vi "DIO read.vi"(8 "error in (no error)":errorcluster, 11 "DIO in":refnum<class "DIO.lvclass">) -> (0 "error out":errorcluster, 2 "read":bool, 3 "DIO out":refnum<class "DIO.lvclass">)   [LabVIEW 2019, in "my FPGA lib.lvlib" / "DIO.lvclass"]
uses:
  DIO.lvclass
  DIO.lvclass/DIO.ctl
  <vilib>/Utility/error.llb/Error Cluster From Error Code.vi
  <vilib>/rvi/errors/niLvFpgaAdjustHostInterfaceError.vi
  <vilib>/rvi/interface/nirviReadWriteControl/nirviReadWriteControl.xnode
  NiFpgaLv.dll
  <vilib>/rvi/interface/Simulation/niFpgaSimulationCallBeginRW.vi
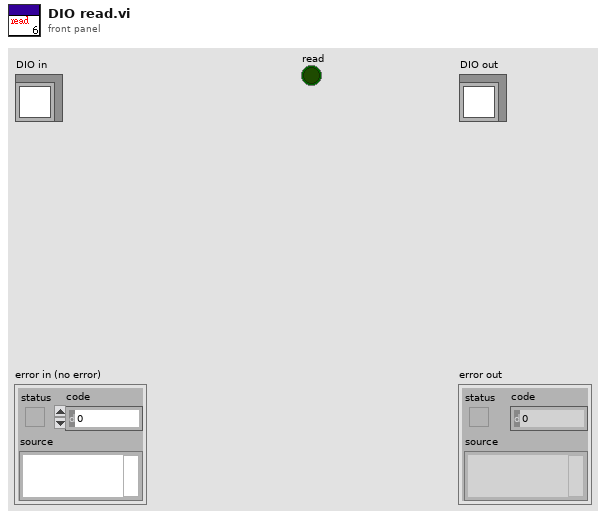
[diagram p1: front panel]
types:
  T1 = typedef "my FPGA lib.lvlib/DIO.lvclass/DIO enum.ctl" = enum16{"US.1", "US.2", "US.3", "US.4", "H.1", "H.2", "H.3", "H.4", "H.5"}
  T2 = typedef "my FPGA lib.lvlib/DIO.lvclass/port.ctl" = enum16{"US", "H."}
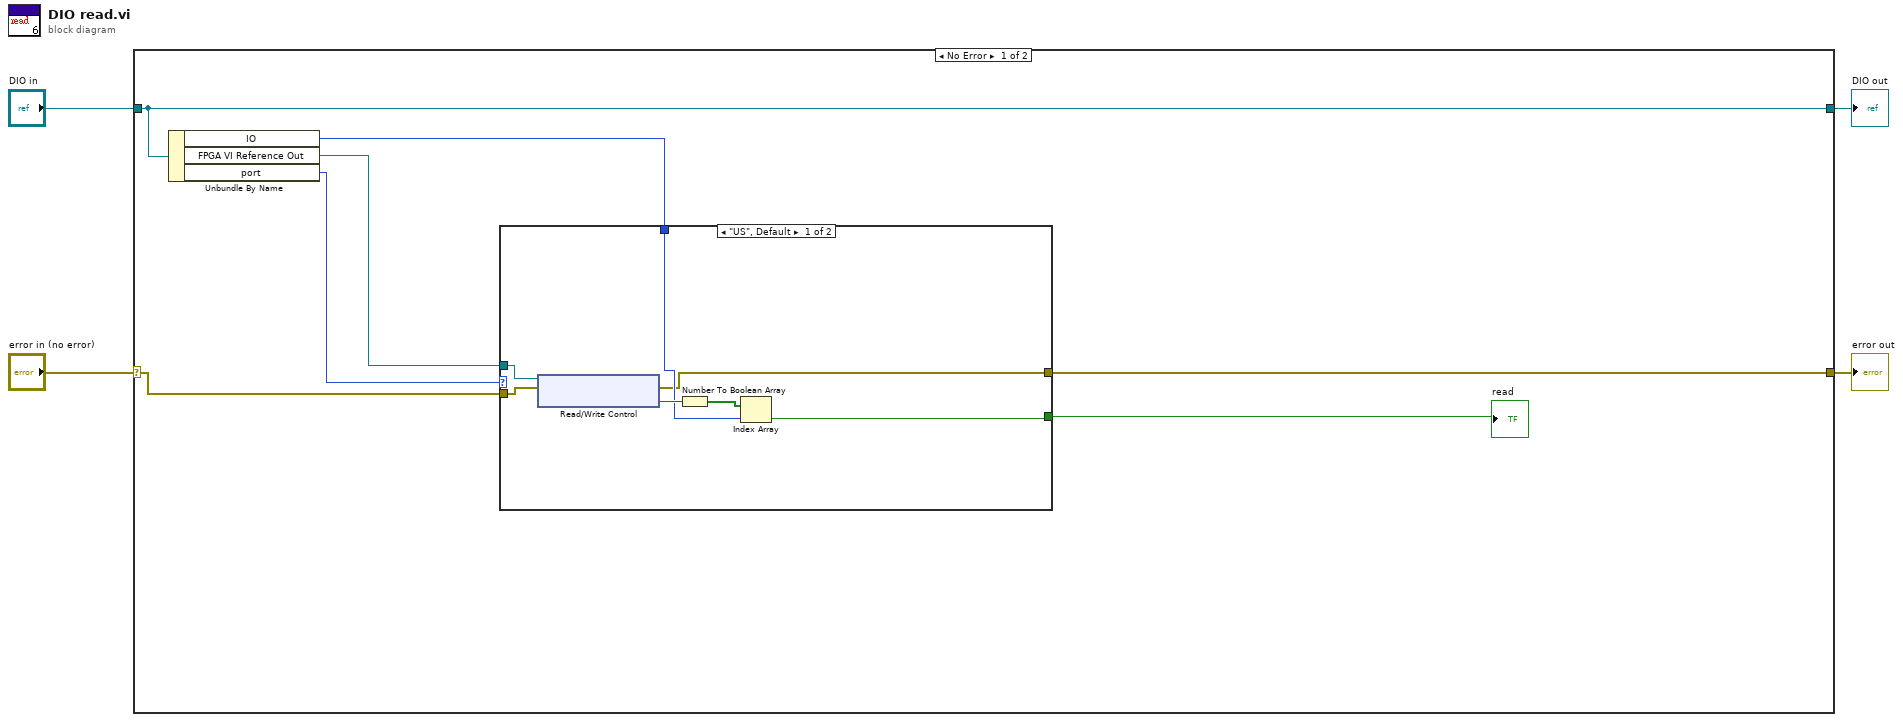
[diagram p0: block diagram]
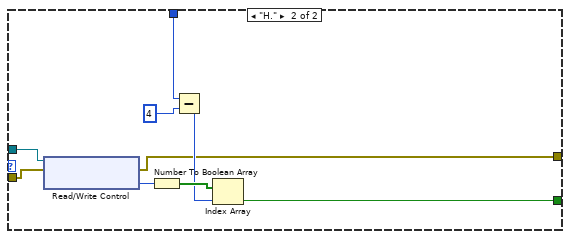
[diagram p2: hidden frame]
diagram:
  n1 = case shown="No Error" "error in (no error)" {
    selector: "error in (no error)" -> [w8 w29]
    tunnel: [w5 w29] -> w3
    tunnel: [w11 w28] -> w1
    tunnel: "DIO in" -> [w11 w28]
    frame No Error {
      n2 = Unbundle By Name(w11) -> ("IO"=w7:T1, "FPGA VI Reference Out"=w9:refnum<k20>, "port"=w10:T2)
      n3 = case shown="\"US\", Default" w10 {
        tunnel: w9 -> [w16 w27]
        tunnel: w8 -> [w15 w26]
        tunnel: w7 -> [w14 w23]
        tunnel: [w13 w20] -> w6
        tunnel: [w12 w19] -> w5
        frame "US", Default {
          n4 = xnode "Read/Write Control"("FPGA VI Reference In"=w16, "error in"=w15) -> ("error out"=w12:errorcluster, "Ultrasonic.io.Read"=w18:u8)  [unwired: 1 out]
          n5 = Number To Boolean Array(number=w18) -> (Boolean array=w17:bool[])
          n6 = Index Array(array=w17, index=w14) -> (element=w13:bool)
        }
        frame "H." {
          n7 = xnode "Read/Write Control"("FPGA VI Reference In"=w27, "error in"=w26) -> ("error out"=w19:errorcluster, "Basic IO Read"=w25:u8)  [unwired: 1 out]
          n8 = Number To Boolean Array(number=w25) -> (Boolean array=w24:bool[])
          n9 = Subtract(x=w23, y=4) -> (x-y=w21:i32)
          n10 = Index Array(array=w24, index=w21) -> (element=w20:bool)
        }
      }
      "read" <- w6
    }
    frame Error {
    }
  }
  "error out" <- w3
  "DIO out" <- w1
